vi "Ouptut_Sound_trace_ph.vi"() -> (5 "Plug in titles":string[](array[string]), 7 "Plug in values":string[](array[string]))   [LabVIEW 2010]
doc: "This VI demonstrates how to output continuous sound using SO Set Num Buffers. This example is available only on Windows."
uses:
  <vilib>/sound/lvsound.llb/Sound Format.ctl
  Globals/Meas_global.vi
  <vilib>/Utility/file.llb/Read From Spreadsheet File (DBL).vi
panel:
  in  "Amplitude":dbl=75.0
  in  "Offset Value":dbl=150.0
  in  "Use default":bool=TRUE
  in  "Trace":dbl[](array[numeric])=array[11200 elements]
  out "size(s)":i32
  in  "Path":path
  out "Waveform Graph":waveform(dbl)(graph)
  out "error out":errorcluster
  in  "Number of buffers":i32(slide)=4 scale=0.0..4.0
  # "Continuous Sound Output Using Buffers"
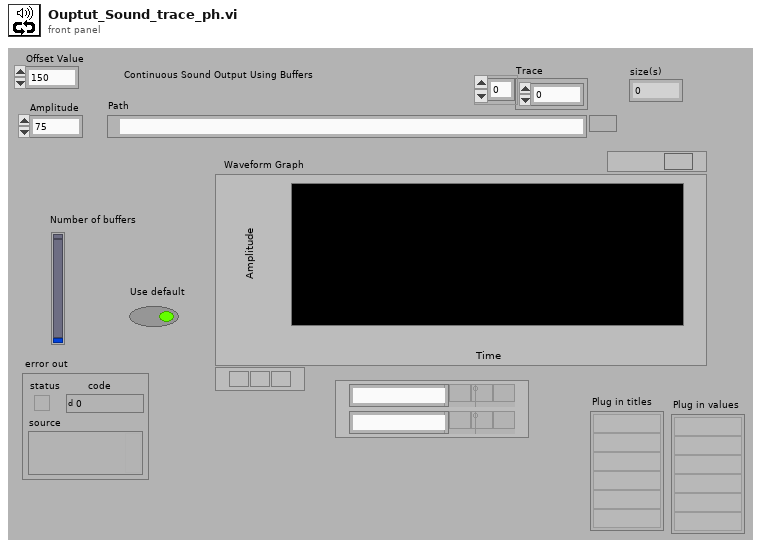
[diagram p1: front panel]
types:
  T1 = typedef "Post_Process.ctl" = enum16{"Take New Data", "Post Process Raw Data File"}
  T2 = typedef "Sound Format.ctl" = cluster{"sound quality":enum16{"mono", "stereo"}, "rate":enum16{"11025", "22050", "44100", "8000"}, "bits per sample":enum16{"8 bit", "16 bit"}}
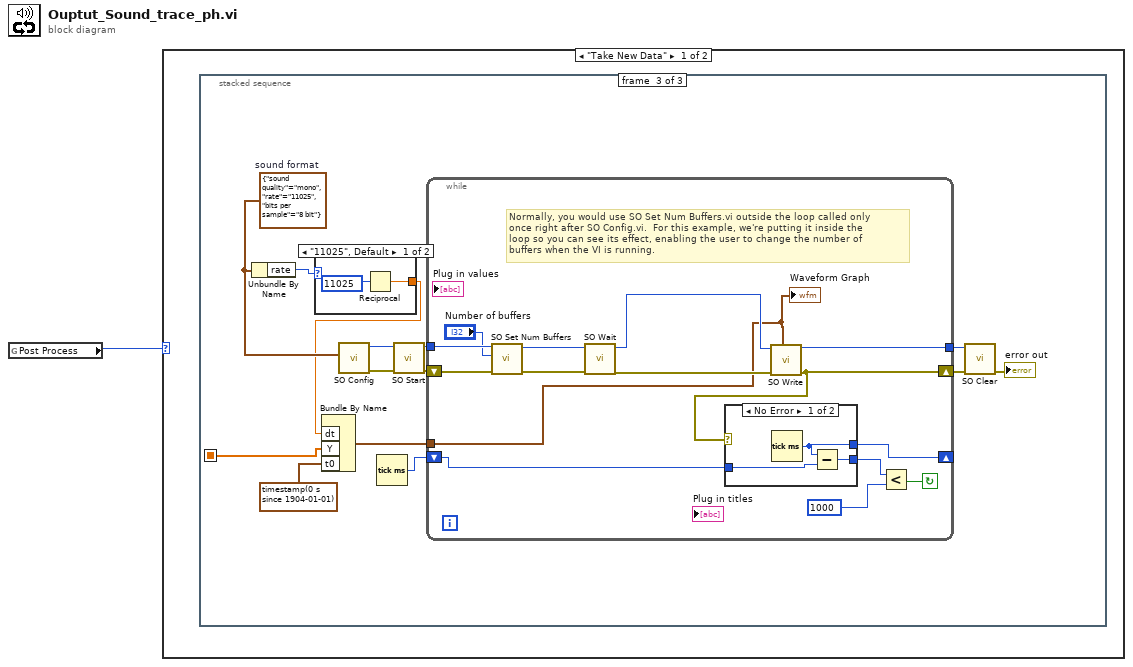
[diagram p0: block diagram]
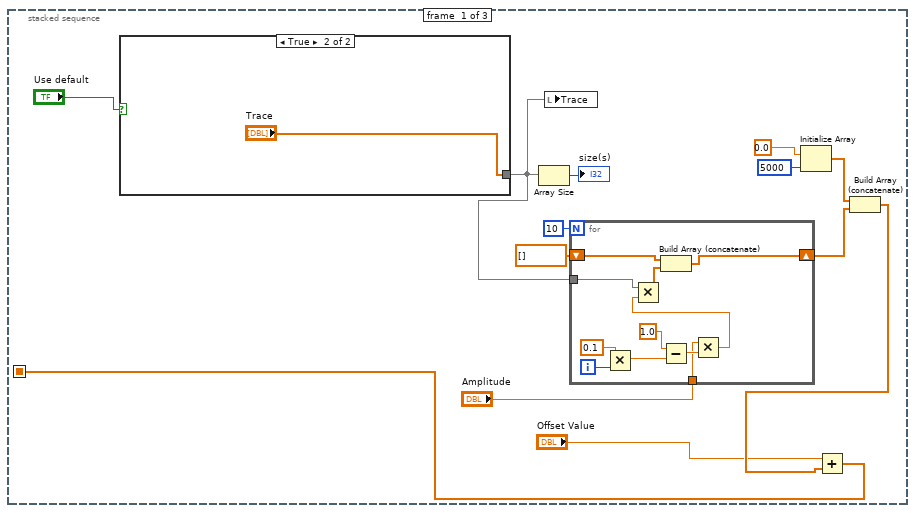
[diagram p2: hidden frame]
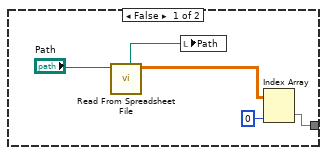
[diagram p3: hidden frame]
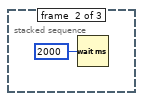
[diagram p4: hidden frame]
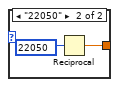
[diagram p6: hidden frame]
diagram:
  n1 = global read "Meas_global.vi" "Post Process"() -> (w1:T1)
  n2 = case shown="\"Take New Data\"" w1 {
    frame "Take New Data" {
      n3 = stacked-sequence {
        seq-local: [w4 _ _] -> [_ _ w34]
        frame #0 {
          n4 = case shown="True" "Use default" {
            tunnel: [w15 "Trace"] -> w6
            frame False {
              n5 = call-poly <vilib>:"Read From Spreadsheet File.vi"("file path (dialog if empty)"="Path") -> ("all rows"=w19:dbl[][], "new file path (Not A Path if cancelled)"=w16:path)  [unwired: 3 in, 6 out]
              n6 = local write "Path"(w16) -> ()
              n7 = Index Array(array=w19, index (col)=0 ("disabled index (col)")) -> (element=w15:dbl[])  [unwired: 1 in]
            }
            frame True {
            }
          }
          n8 = Array Size(array=w6) -> (size(s)=→"size(s)":i32)
          n9 = local write "Trace"(w6) -> ()
          n10 = for {
            N: 10 -> [_]
            shift-right: [w30] -> w7
            shift-left: dbl[] [] -> [w31]
            tunnel: w6 -> [w25]
            tunnel: "Amplitude" -> [w21]
            i -> [w29]
            n11 = Multiply(x=0.1, y=w29) -> (x*y=w26:dbl)
            n12 = Subtract(x=1.0, y=w26) -> (x-y=w23:dbl)
            n13 = Multiply(x=w21, y=w23) -> (x*y=w22:dbl)
            n14 = Multiply(x=w25, y=w22) -> (x*y=w24:dbl[])
            n15 = Build Array (concatenate)(w31, w24) -> (w30:dbl[])
          }
          n16 = Initialize Array(0.0 ("x"), 5000 ("dimension size")) -> (w8:dbl[])
          n17 = Build Array (concatenate)(w8, w7) -> (w5:dbl[])
          n18 = Add(x="Offset Value", y=w5) -> (x+y=w4:dbl[])
        }
        frame #1 {
          n19 = Wait (ms)(milliseconds to wait=u32 2000) -> ()  [unwired: 1 out]
        }
        frame #2 {
          w39 = T2 {"sound quality"=enum."mono", "rate"=enum."11025", "bits per sample"=enum."8 bit"}  # sound format
          n20 = Unbundle By Name(w39) -> ("rate"=w38:enum16{"11025", "22050", "44100", "8000"})
          n21 = case shown="\"11025\", Default" w38 {
            tunnel: [w66 w68] -> w36
            frame "11025", Default {
              n22 = Reciprocal(x=11025) -> (1/x=w66:dbl)
            }
            frame "22050" {
              n23 = Reciprocal(x=22050) -> (1/x=w68:dbl)
            }
          }
          n24 = Bundle By Name("dt"=w36, "Y"=w34, "t0"=timestamp(0 s since 1904-01-01)) -> (w35:waveform(dbl))  [unwired: 1 out]
          n25 = call <vilib>:"SO Config.vi"("sound format"=w39) -> ("error out"=w45:errorcluster, "task ID out"=w46:u32)  [unwired: 1 in, 8 out]
          n26 = Tick Count (ms)() -> (millisecond timer value=w33:u32)
          n27 = call <vilib>:"SO Start.vi"("error in (no error)"=w45, "task ID in"=w46) -> ("error out"=w44:errorcluster, "task ID out"=w43:u32)  [unwired: 8 out]
          n28 = while {
            shift-right: [w52] -> w42
            shift-left: w44 -> [w60]
            tunnel: w43 -> [w58]
            tunnel: [w55] -> w41
            tunnel: w35 -> [w53]
            shift-right: [w50] -> _
            shift-left: w33 -> [w51]
            stop <- w47 continue-if-true
            # "Normally, you would use SO Set Num Buffers.vi outside the loop called only\nonce right after SO Config.vi.  For this example, we're putting it inside the\nloop so you can see its effect, enabling the user to change the number of\nbuffers when the VI is running."
            n29 = call <vilib>:"SO Set Num Buffers.vi"("error in (no error)"=w60, "number of buffers"="Number of buffers", "task ID in"=w58) -> ("error out"=w59:errorcluster, "task ID out"=w57:u32)  [unwired: 7 out]
            n30 = call <vilib>:"SO Wait.vi"("error in (no error)"=w59, "task ID in"=w57) -> ("error out"=w54:errorcluster, "task ID out"=w61:u32)  [unwired: 8 out]
            n31 = call <vilib>:"SO Write.vi"("mono 8-bit"=w53, "error in (no error)"=w54, "task ID in"=w61) -> ("error out"=w52:errorcluster, "task ID out"=w55:u32)  [unwired: 3 in, 4 out]
            n32 = case shown="No Error" w52 {
              tunnel: w51 -> [w64 w65]
              tunnel: [w63 w65] -> w50
              tunnel: [w62 w65] -> w49
              frame No Error {
                n33 = Tick Count (ms)() -> (millisecond timer value=w63:u32)
                n34 = Subtract(x=w63, y=w64) -> (x-y=w62:u32)
              }
              frame Error {
              }
            }
            n35 = Less?(x=w49, y=u32 1000) -> (x < y?=w47:bool)
            "Waveform Graph" <- w53
          }
          n36 = call <vilib>:"SO Clear.vi"("error in (no error)"=w42, "task ID in"=w41) -> ("error out"=→"error out":errorcluster)  [unwired: 9 out]
        }
      }
    }
    frame "Post Process Raw Data File" {
    }
  }
